vi "parse file string.vi"(8 "error in":errorcluster, 11 "data string":string) -> (0 "error out":errorcluster, 3 "file format":T1)   [LabVIEW 2013, in "PLConfigurationSerializer.lvlib"]
uses:
  PLConfigurationSerializer.lvlib
  file format.ctl
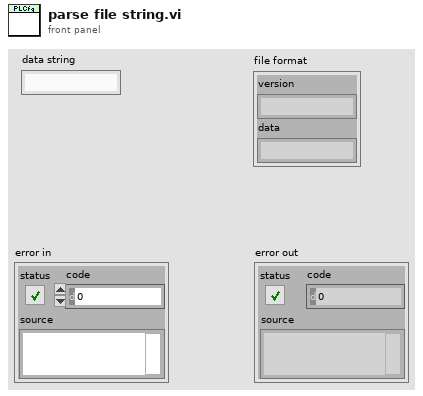
[diagram p1: front panel]
types:
  T1 = typedef "PLConfigurationSerializer.lvlib/file format.ctl" = cluster{"version":string, "data":string}
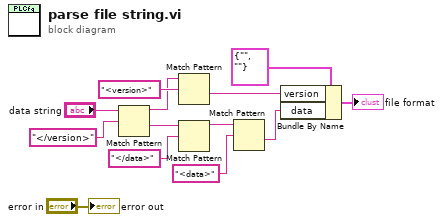
[diagram p0: block diagram]
diagram:
  n1 = Match Pattern(string="data string", regular expression="</version>") -> (before substring=w8:string, after substring=w1:string)  [unwired: 1 in, 2 out]
  n2 = Match Pattern(string=w8, regular expression="<version>") -> (after substring=w4:string)  [unwired: 1 in, 3 out]
  n3 = Match Pattern(string=w1, regular expression="</data>") -> (before substring=w2:string)  [unwired: 1 in, 3 out]
  n4 = Match Pattern(string=w2, regular expression="<data>") -> (after substring=w3:string)  [unwired: 1 in, 3 out]
  n5 = Bundle By Name(cluster=T1 {"version"="", "data"=""} ("file format"), "version"=w4, "data"=w3) -> (→"file format":T1)
  "error out" <- "error in"
